vi "Notatnik.vi"() -> ()   [LabVIEW 2020]
uses:
  #typeDef_ProgramData.ctl
panel:
  out "New":bool
  out "Save":bool
  in  "Sortuj":bool
  in  "Jump Button":bool
  in  "Listbox":i32[](listbox)
  in  "Delete Button":bool
  in  "Save Button":bool
  in  "Open Button":bool
  in  "New Button":bool
  in  "Note":string
  in  "Title":string
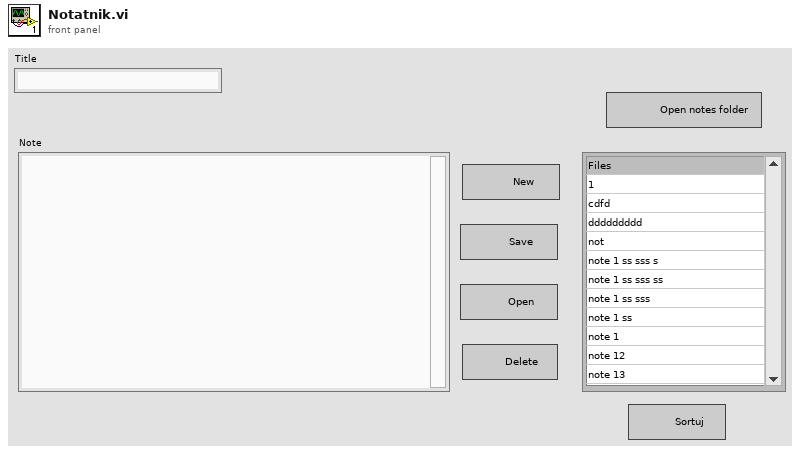
[diagram p1: front panel]
types:
  T1 = typedef "#typeDef_ProgramData.ctl" = cluster{"Tytuły":string[], "Folder":path, "Data/tytul":cluster{"Data":timestamp, "Tytuł":string}[], "Ostatni index":i32, "Title":string, "Note":string}
  T2 = cluster{"Shift":bool, "Ctrl":bool, "Alt":bool, "Cmd":bool, "Opt":bool}
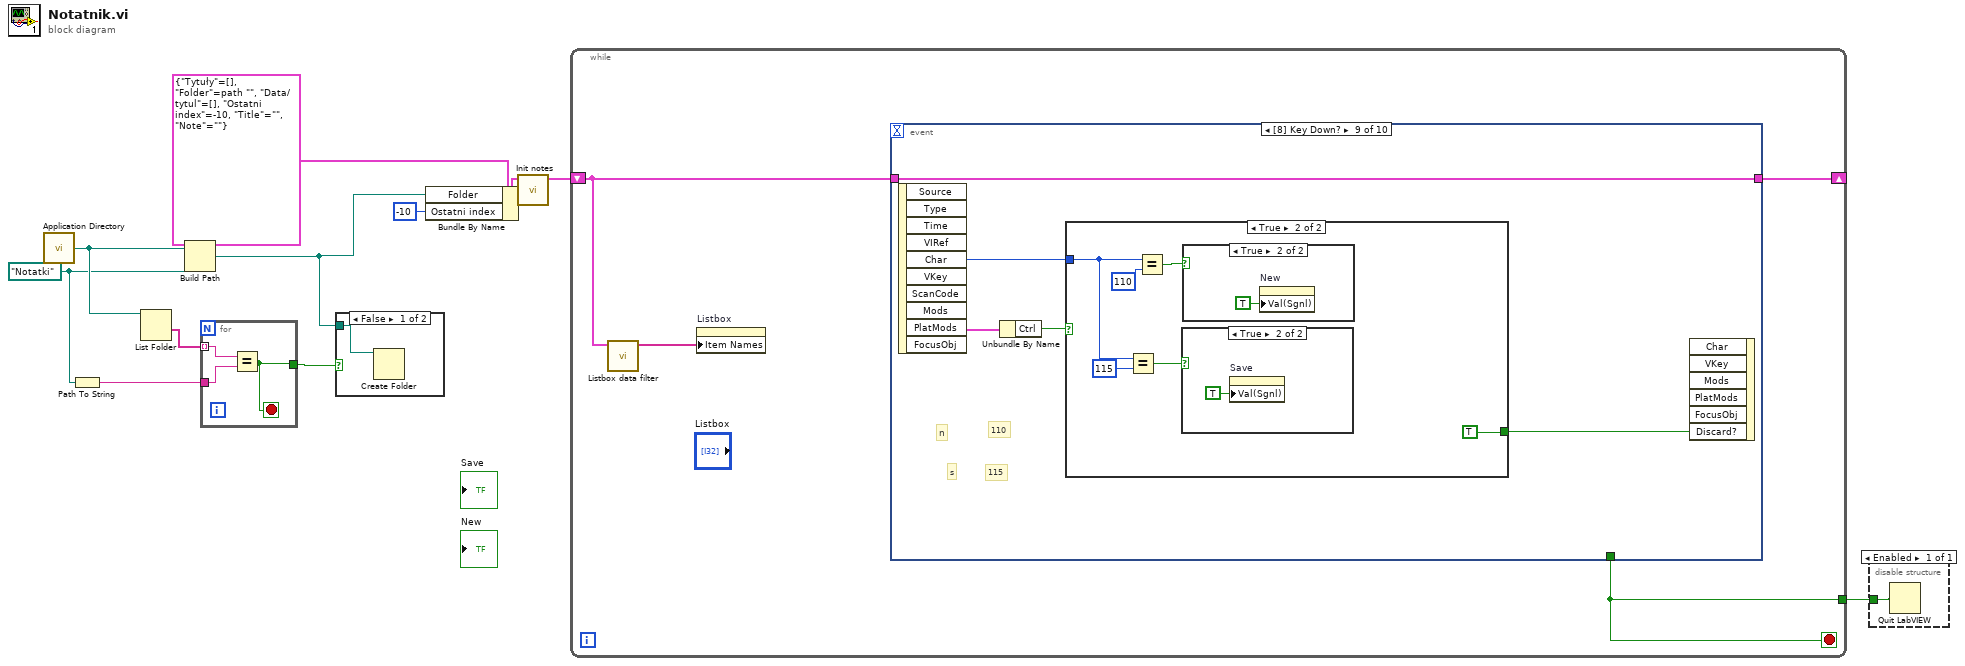
[diagram p0: block diagram]
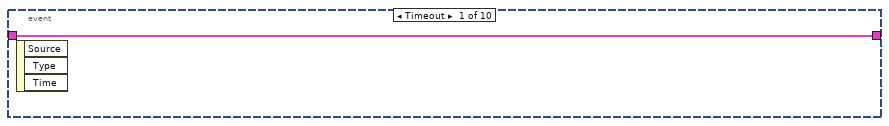
[diagram p3: hidden frame]
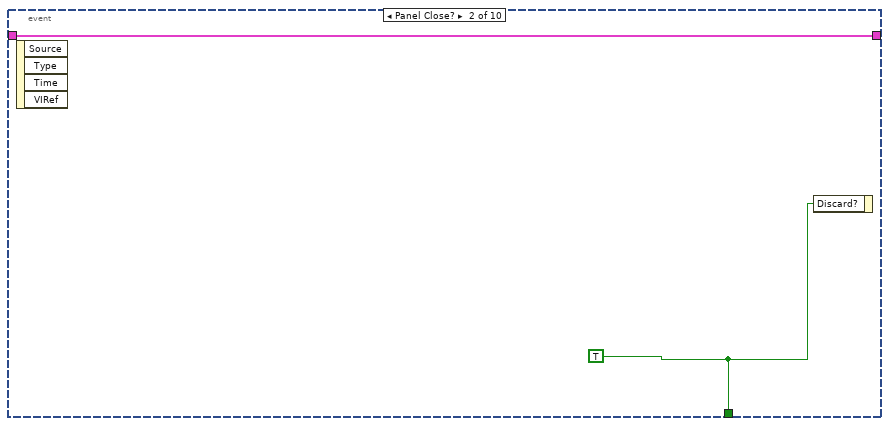
[diagram p4: hidden frame]
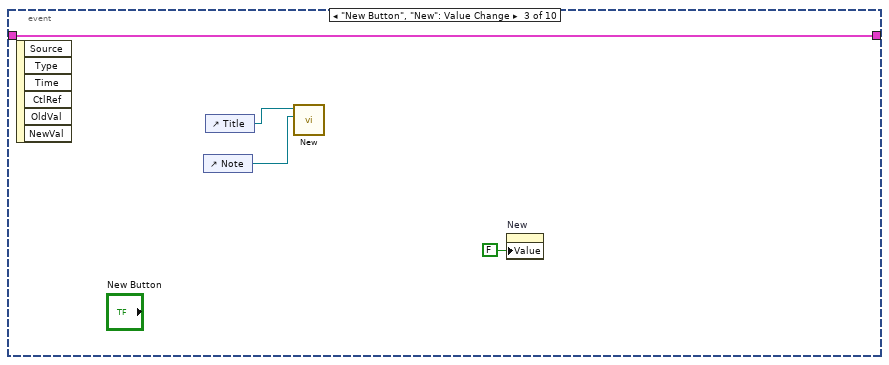
[diagram p5: hidden frame]
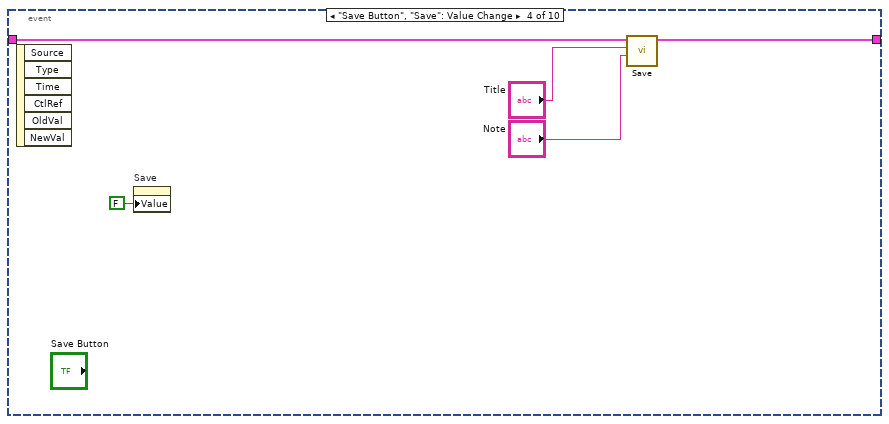
[diagram p6: hidden frame]
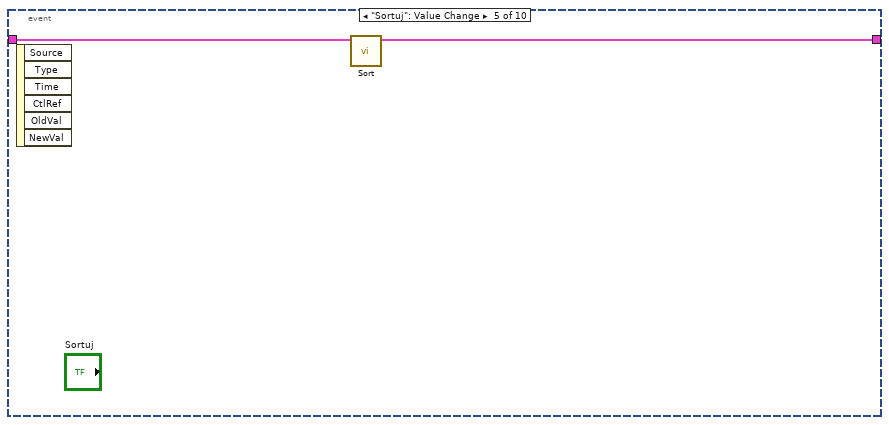
[diagram p7: hidden frame]
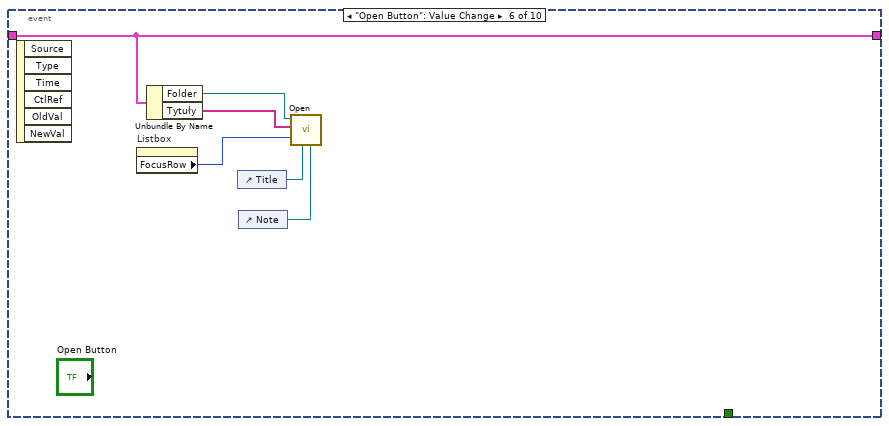
[diagram p8: hidden frame]
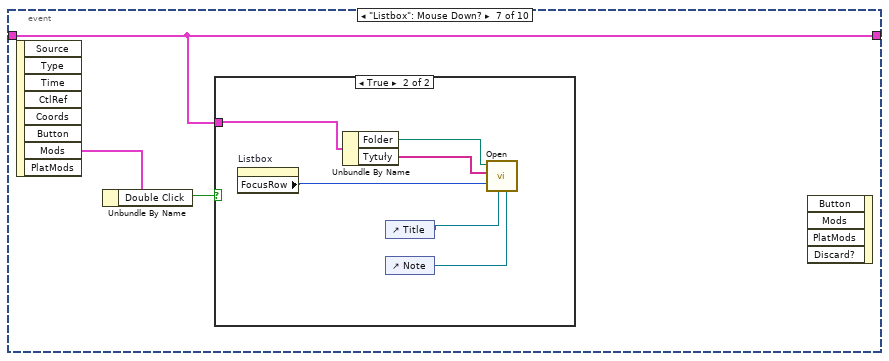
[diagram p9: hidden frame]
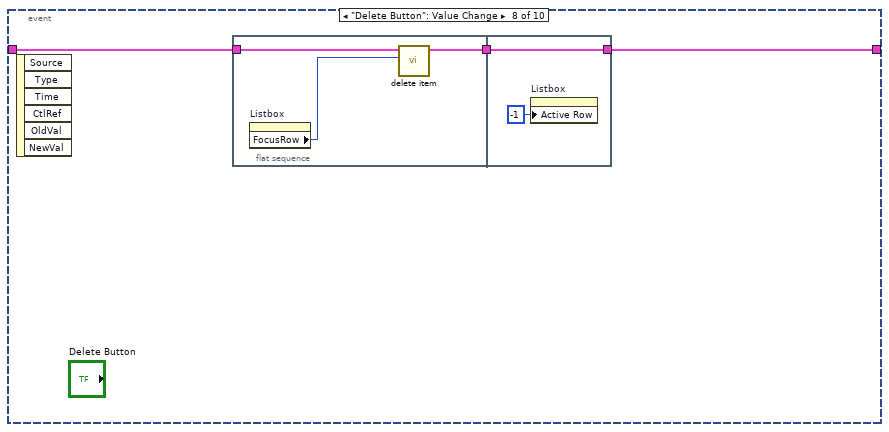
[diagram p11: hidden frame]
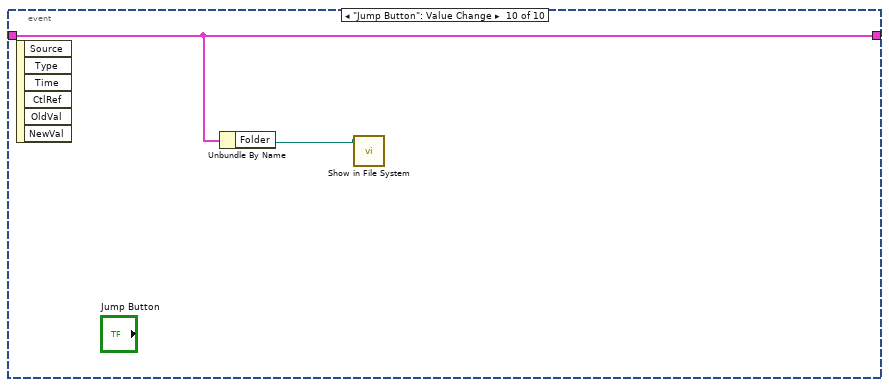
[diagram p15: hidden frame]
diagram:
  w7 = path "Notatki" ("name or relative path")
  n1 = call <vilib>:"Application Directory.vi"() -> ("Application Directory"=w9:path)
  n2 = Path To String(path=w7) -> (string=w6:string)
  n3 = List Folder(path=w9) -> (folder names=w8:string[])  [unwired: 3 in, 3 out]
  n4 = Build Path(base path=w9, name or relative path=w7) -> (appended path=w4:path)
  n5 = for {
    tunnel: w8 -> [w14] mode=indexing
    tunnel: w6 -> [w13]
    tunnel: [w12] -> w5
    stop <- w12 stop-if-true
    n6 = Equal?(x=w14, y=w13) -> (x = y?=w12:bool)
  }
  n7 = case shown="False" w5 {
    tunnel: w4 -> [w15 _]
    frame False {
      n8 = Create Folder(path (use dialog)=w15) -> ()  [unwired: 2 in, 3 out]
    }
    frame True {
    }
  }
  n9 = Bundle By Name(cluster=T1 {"Tytuły"=[], "Folder"=path "", "Data/tytul"=[], "Ostatni index"=-10, "Title"="", "Note"=""}, "Folder"=w4, "Ostatni index"=-10) -> (w2:T1)
  n10 = call "Init notes.vi"(11:w2) -> (3:w3:T1)  [unwired: 10 in]
  n11 = while {
    shift-right: [w19] -> _
    shift-left: w3 -> [w16]
    tunnel: [w18] -> w10
    stop <- w18 stop-if-true
    n12 = call "Listbox data filter.vi"("ProgramData"=w16) -> ("Array"=w17:string[])  [unwired: 10 in]
    n13 = property on="Listbox" class="LstBox (strict)"("Item Names"=w17) -> ()  [unwired: 2 in, 2 out]
    n14 = event shown="[8] Key Down?" {
      selector: _ -> [_ _ _ _ _ _ _ _ _ _]
      dyn-events: _ -> [_ _ _ _ _ _ _ _ _ _]
      timeout: _ -> [_ _ _ _ _ _ _ _ _ _]
      tunnel: [_ w21 _ _ _ _ _ _ _ _] -> w18
      tunnel: [w20 w22 w25 w31 w32 w39 w42 w51 w61 w71] -> w19
      tunnel: w16 -> [w20 w22 w25 w29 w33 w39 w42 w50 w61 w71]
      event Timeout {
        n15 = event-data() -> ()  [unwired: 1 in, 3 out]
      }
      event Panel Close? {
        w21 = TRUE
        n16 = event-data() -> ()  [unwired: 1 in, 4 out]
        n17 = event-data("Discard?"=w21) -> ()  [unwired: 1 in, 1 out]
      }
      event "New Button", "New": Value Change {
        n18 = event-data() -> ()  [unwired: 1 in, 6 out]
        n19 = control-ref of="Note"() -> (w23:refnum<vi>)
        n20 = control-ref of="Title"() -> (w24:refnum<vi>)
        n21 = call "New.vi"("note refnum"=w23, "title refnum"=w24) -> ()  [unwired: 10 in]
        n22 = property on="New" class="Bool (strict)"("Value"=FALSE ("New")) -> ()  [unwired: 2 in, 2 out]
      }
      event "Save Button", "Save": Value Change {
        n23 = event-data() -> ()  [unwired: 1 in, 6 out]
        n24 = property on="Save" class="Bool (strict)"("Value"=FALSE ("Save")) -> ()  [unwired: 2 in, 2 out]
        n25 = call "Save.vi"("Notatka"="Note", "Tytuł"="Title", "ProgramData in"=w29) -> ("ProgramData out"=w31:T1)  [unwired: 8 in]
      }
      event "Sortuj": Value Change {
        n26 = event-data() -> ()  [unwired: 1 in, 6 out]
        n27 = call "Sort.vi"("ProgramData"=w33) -> ("ProgramData Exit"=w32:T1)  [unwired: 10 in]
      }
      event "Open Button": Value Change {
        n28 = event-data() -> ()  [unwired: 1 in, 6 out]
        n29 = property on="Listbox" class="LstBox (strict)"() -> ("FocusRow"=w35:i32)  [unwired: 2 in, 2 out]
        n30 = Unbundle By Name(w39) -> ("Folder"=w36:path, "Tytuły"=w34:string[])
        n31 = control-ref of="Title"() -> (w38:refnum<vi>)
        n32 = control-ref of="Note"() -> (w37:refnum<vi>)
        n33 = call "Open.vi"("Notatka refnum"=w37, "Tytul refnum"=w38, "Active Row"=w35, "Tytuły"=w34, "Folder"=w36) -> ()  [unwired: 7 in]
      }
      event "Listbox": Mouse Down? {
        n34 = event-data() -> ("Mods"=w41:cluster{"Double Click":bool, "Menu Key":bool})  [unwired: 1 in, 7 out]
        n35 = Unbundle By Name(w41) -> ("Double Click"=w40:bool)
        n36 = case shown="True" w40 {
          tunnel: w42 -> [_ w46]
          frame False {
          }
          frame True {
            n37 = property on="Listbox" class="LstBox (strict)"() -> ("FocusRow"=w45:i32)  [unwired: 2 in, 2 out]
            n38 = Unbundle By Name(w46) -> ("Folder"=w47:path, "Tytuły"=w48:string[])
            n39 = control-ref of="Title"() -> (w43:refnum<vi>)
            n40 = control-ref of="Note"() -> (w44:refnum<vi>)
            n41 = call "Open.vi"("Notatka refnum"=w44, "Tytul refnum"=w43, "Active Row"=w45, "Tytuły"=w48, "Folder"=w47) -> ()  [unwired: 7 in]
          }
        }
        n42 = event-data() -> ()  [unwired: 5 in, 1 out]
      }
      event "Delete Button": Value Change {
        n43 = event-data() -> ()  [unwired: 1 in, 6 out]
        n44 = flat-sequence {
          tunnel: w50 -> [w52]
          tunnel: [w53] -> w49
          tunnel: [w56] -> w51
          tunnel: w49 -> [w56]
          frame #0 {
            n45 = property on="Listbox" class="LstBox (strict)"() -> ("FocusRow"=w54:i32)  [unwired: 2 in, 2 out]
            n46 = call "delete item.vi"("Index"=w54, "ProgramData in"=w52) -> ("ProgramData out"=w53:T1)  [unwired: 9 in]
          }
          frame #1 {
            n47 = property on="Listbox" class="LstBox (strict)"("Active Row"=-1 ("Focus Row")) -> ()  [unwired: 2 in, 2 out]
          }
        }
      }
      event Key Down? {
        # "115"
        # "110"
        # "s"
        # "n"
        n48 = event-data() -> ("Char"=w59:i16, "PlatMods"=w60:T2)  [unwired: 1 in, 8 out]
        n49 = Unbundle By Name(w60) -> ("Ctrl"=w58:bool)
        n50 = case shown="True" w58 {
          tunnel: w59 -> [_ w65]
          tunnel: [_ TRUE] -> w57
          frame False {
          }
          frame True {
            n51 = Equal?(x=w65, y=i16 115) -> (x = y?=w63:bool)
            n52 = Equal?(x=w65, y=i16 110) -> (x = y?=w67:bool)
            n53 = case shown="True" w63 {
              frame False {
              }
              frame True {
                n54 = property on="Save" class="Bool (strict)"("Val(Sgnl)"=TRUE ("Value (Signaling)")) -> ()  [unwired: 2 in, 2 out]
              }
            }
            n55 = case shown="True" w67 {
              frame False {
              }
              frame True {
                n56 = property on="New" class="Bool (strict)"("Val(Sgnl)"=TRUE ("Value (Signaling)")) -> ()  [unwired: 2 in, 2 out]
              }
            }
          }
        }
        n57 = event-data("Discard?"=w57) -> ()  [unwired: 6 in, 1 out]
      }
      event "Jump Button": Value Change {
        n58 = event-data() -> ()  [unwired: 1 in, 6 out]
        n59 = Unbundle By Name(w71) -> ("Folder"=w70:path)
        n60 = call <vilib>:"Show in File System.vi"("file or directory path"=w70) -> ()  [unwired: 10 in, 1 out]
      }
    }
  }
  n61 = disable-structure shown="Enabled" {
    disable-tunnel: w10 -> [w72]
    frame Enabled {
      n62 = Quit LabVIEW(quit? (T)=w72) -> ()
    }
  }
